vi "Serialize.vi"(8 "error in (no error)":errorcluster, 11 "ConverterBase in":refnum<class "ClassConverter.lvclass">) -> (0 "error out":errorcluster, 2 "JSON":string, 3 "ConverterBase out":refnum<class "ClassConverter.lvclass">)   [LabVIEW 2017, in "ClassConverter.lvclass"]
uses:
  ClassConverter.lvclass
  Helpers/DirectoryMetadata/DirectoryMetadata.lvclass
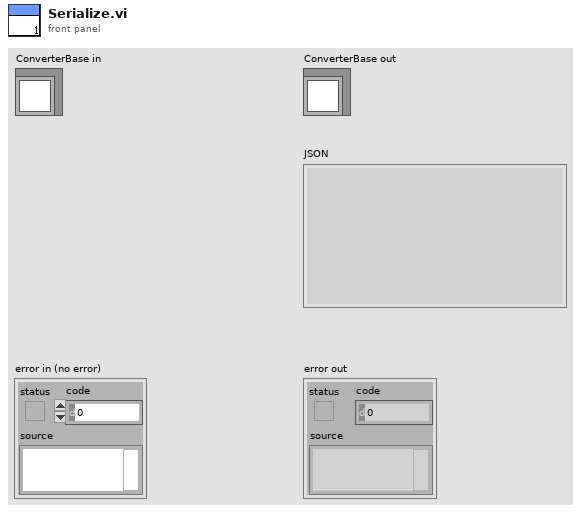
[diagram p1: front panel]
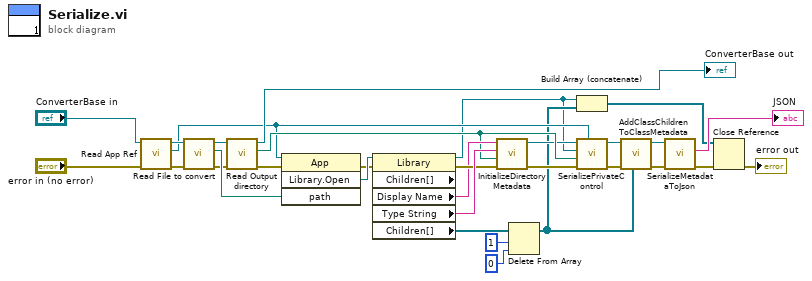
[diagram p0: block diagram]
diagram:
  n1 = call-dynamic "Read App Ref.vi"("error in (no error)"="error in (no error)", "FileConverterBase in"="ConverterBase in") -> ("error out"=w20:errorcluster, "App Ref"=w14:refnum<vi>, "FileConverterBase out"=w26:refnum<class "ClassConverter.lvclass">)  [unwired: 7 in]
  n2 = call-dynamic "Read File to convert.vi"("error in (no error)"=w20, "FileConverterBase in"=w26) -> ("error out"=w17:errorcluster, "Input File Path"=w25:path, "FileConverterBase out"=w19:refnum<class "ClassConverter.lvclass">)  [unwired: 7 in]
  n3 = call-dynamic "Read Output directory.vi"("error in (no error)"=w17, "FileConverterBase in"=w19) -> ("error out"=w16:errorcluster, "Output JSON File Path"=w15:path, "FileConverterBase out"=→"ConverterBase out":refnum<class "ClassConverter.lvclass">)  [unwired: 7 in]
  n4 = invoke class="App" method="Library.Open"(reference=w14, error in=w16, "path"=w25) -> (error out=w30:errorcluster, "Open Library"=w31:refnum<vi>)  [unwired: 1 in, 2 out]
  n5 = property class="Library" props=["Children[]", "Display Name", "Type String", "Children[]"](reference=w31, error in=w30) -> (reference out=w3:refnum<vi>, error out=w27:errorcluster, "Display Name"=w24:string, "Type String"=w29:string, "Children[]"=w1:refnum<vi>[])  [unwired: 1 out]
  n6 = call "InitializeDirectoryMetadata.vi"("Error in"=w27, "Path"=w15, "Type"=w29, "ID"=w24) -> ("Error out"=w9:errorcluster, "DirectoryMetadata instance"=w13:refnum<data-value>)  [unwired: 6 in]
  n7 = Delete From Array(array=w1, length=1, index=0) -> (array with subset deleted=w4:refnum<vi>[])  [unwired: 1 out]
  n8 = Build Array (concatenate)(w3, w4) -> (w2:refnum<vi>[])
  n9 = call "SerializePrivateControl.vi"("App Ref"=w14, "error in (no error)"=w9, "Output JSON File Path"=w15, "Library"=w3, "Root in"=w13) -> ("error out"=w7:errorcluster, "Root out"=w12:refnum<data-value>)  [unwired: 5 in]
  n10 = call "AddClassChildrenToClassMetadata.vi"("Children[]"=w4, "error in"=w7, "ClassMetadata instance"=w12) -> ("error out"=w6:errorcluster, "ClassMetadata instance out"=w28:refnum<data-value>)  [unwired: 7 in]
  n11 = call "SerializeMetadataToJson.vi"("error in (no error)"=w6, "head in"=w28) -> ("error out"=w8:errorcluster, "Serialized String"=→"JSON":string)  [unwired: 7 in, 1 out]
  n12 = Close Reference(reference=w2, error in (no error)=w8) -> (error out=→"error out":errorcluster)
